vi "main-test.vi"() -> ()   [LabVIEW 2018]
uses:
  Lib/Korad/Korad KA3305P.lvlib
  Lib/Korad/Channels.ctl
  Lib/Korad/Out stat.ctl
  Lib/Korad/Tracking.ctl
  Lib/Korad/Status.ctl
panel:
  out "Status 2":T1
  out "Status":string
  in  "Tracking":T2
  out "Iset?":dbl
  out "sIset?":string
  out "Vset?":dbl
  out "sVset?":string
  in  "Delay (30ms)":dbl=0.03 format="%#_13g"
  in  "OUT stat":T3
  out "error out":errorcluster
  in  "Value (0-5)":dbl min=0.0 max=5.0 format="%#.3g"
  in  "Value (0-30)":dbl min=0.0 max=30.0
  in  "Channel":T4
  out "length":i32
  out "data out":string
  in  "data":string
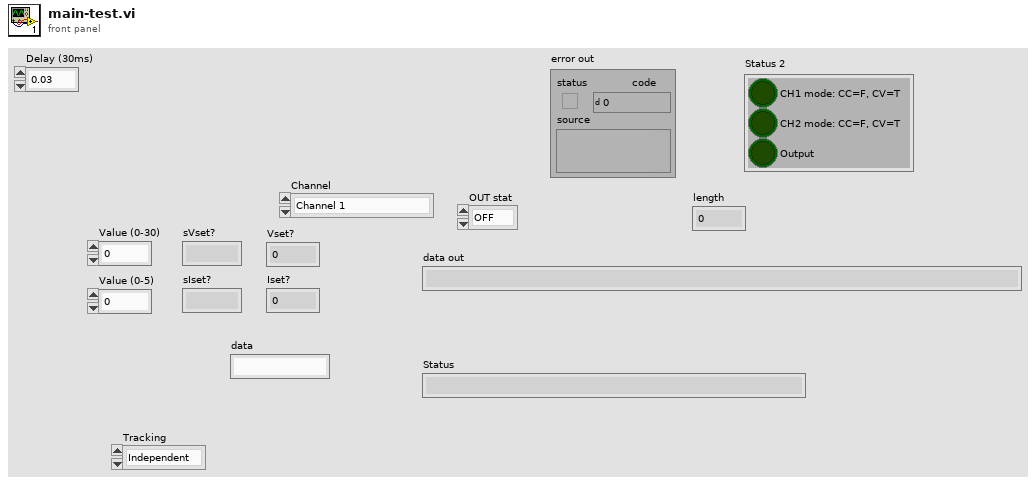
[diagram p1: front panel]
types:
  T1 = typedef "Korad KA3305P.lvlib/Status.ctl" = cluster{"CH1 mode: CC=F, CV=T":bool, "CH2 mode: CC=F, CV=T":bool, "Output":bool}
  T2 = typedef "Korad KA3305P.lvlib/Tracking.ctl" = enum16{"Independent", "Serial", "Parallel"}
  T3 = typedef "Korad KA3305P.lvlib/Out stat.ctl" = enum16{"OFF", "ON"}
  T4 = typedef "Korad KA3305P.lvlib/Channels.ctl" = enum16{"Channel 1", "Channel 2"}
  T5 = typedef "Korad KA3305P.lvlib/Reference.ctl" = cluster{"refnum":refnum<visa-resource-name>, "timestamp":timestamp, "Delay":dbl}
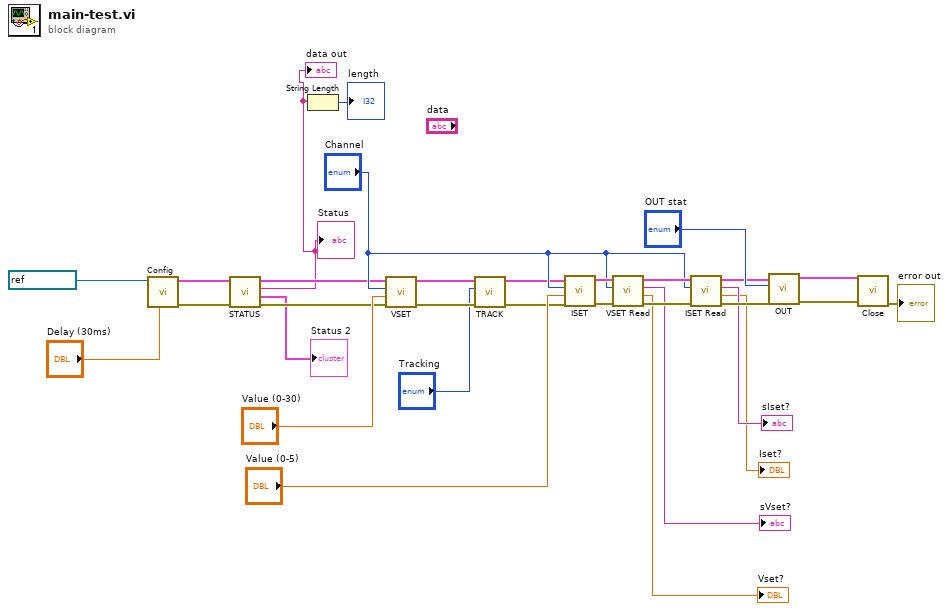
[diagram p0: block diagram]
diagram:
  n1 = call "Config.vi"("Delay (30ms)"="Delay (30ms)", "COM PPORT"=refnum<visa-resource-name> "COM18") -> ("error out"=w29:errorcluster, "refnum out"=w4:T5)  [unwired: 8 in]
  n2 = call "STATUS.vi"("error in (no error)"=w29, "refnum in"=w4) -> ("error out"=w5:errorcluster, "Status"=→"Status 2":T1, "data out"=w2:string, "refnum out"=w3:T5)  [unwired: 5 in, 1 out]
  "data out" <- w2
  "Status" <- w2
  n3 = String Length(string=w2) -> (length=→"length":i32)
  n4 = call "VSET.vi"("error in (no error)"=w5, "Value (0-30)"="Value (0-30)", "Channel"="Channel", "refnum in"=w3) -> ("error out"=w26:errorcluster, "refnum out"=w8:T5)  [unwired: 5 in, 1 out]
  n5 = call "TRACK.vi"("error in (no error)"=w26, "Tracking"="Tracking", "refnum in"=w8) -> ("error out"=w9:errorcluster, "refnum out"=w7:T5)  [unwired: 6 in, 1 out]
  n6 = call "ISET.vi"("error in (no error)"=w9, "Value (0-5)"="Value (0-5)", "Channel"="Channel", "refnum in"=w7) -> ("error out"=w21:errorcluster, "refnum out"=w18:T5)  [unwired: 5 in, 1 out]
  n7 = call "VSET Read.vi"("error in (no error)"=w21, "Channel"="Channel", "refnum in"=w18) -> ("error out"=w19:errorcluster, "Vset?"=→"Vset?":dbl, "sVset"=→"sVset?":string, "refnum out"=w14:T5)  [unwired: 4 in, 1 out]
  n8 = call "ISET Read.vi"("error in (no error)"=w19, "Channel"="Channel", "refnum in"=w14) -> ("error out"=w15:errorcluster, "Iset?"=→"Iset?":dbl, "sIset"=→"sIset?":string, "refnum out"=w13:T5)  [unwired: 4 in, 1 out]
  n9 = call "OUT.vi"("error in (no error)"=w15, "OUT stat"="OUT stat", "refnum in"=w13) -> ("error out"=w23:errorcluster, "refnum out"=w24:T5)  [unwired: 6 in, 1 out]
  n10 = call "Close.vi"("error in (no error)"=w23, "refnum in"=w24) -> ("error out"=→"error out":errorcluster)  [unwired: 9 in]
